vi "test - clear JKI String Queue Error.vi"(8 "error in (no error)":errorcluster, 11 "TestCase in":refnum<class "testcase-Basic-Function.lvclass">) -> (0 "error out":errorcluster, 3 "TestCase out":refnum<class "testcase-Basic-Function.lvclass">)   [LabVIEW 2017, in "testcase-Basic-Function.lvclass"]
uses:
  testcase-Basic-Function.lvclass
  161a5074-68cb-42ac-bbbd-290e101bf616.vi
  src/user.lib/_NEVSTOP/Communicable State Machine(CSM)/AdvanceAPI/CSM - Revert Arguments-Safe String.vi
  src/user.lib/_NEVSTOP/Communicable State Machine(CSM)/_Support/Common/Trim Single line Text.vi
  src/user.lib/_NEVSTOP/Communicable State Machine(CSM)/AdvanceAPI/CSM - Make String Arguments Safe.vi
  src/user.lib/_NEVSTOP/Communicable State Machine(CSM)/AdvanceAPI/CSM - Break Down Multiple States String.vi
  src/user.lib/_NEVSTOP/Communicable State Machine(CSM)/AdvanceAPI/CSM - Compact Multiple States.vi
  src/user.lib/_NEVSTOP/Communicable State Machine(CSM)/AdvanceAPI/CSM - Keywords.vi
  <vilib>/addons/_JKI Toolkits/VI Tester/TestCase.llb/TestCase.lvclass
  src/user.lib/_NEVSTOP/Communicable State Machine(CSM)/Communicable State Machine.lvlib
  C:/Program Files (x86)/National Instruments/LabVIEW 2017/vi.lib/addons/_JKI Toolkits/VI Tester/TestCase.llb/TestCase.lvclass
panel:
  out "error in CSM":errorcluster
  in  "x":bool
  out "error for return":errorcluster
  out "State History":string
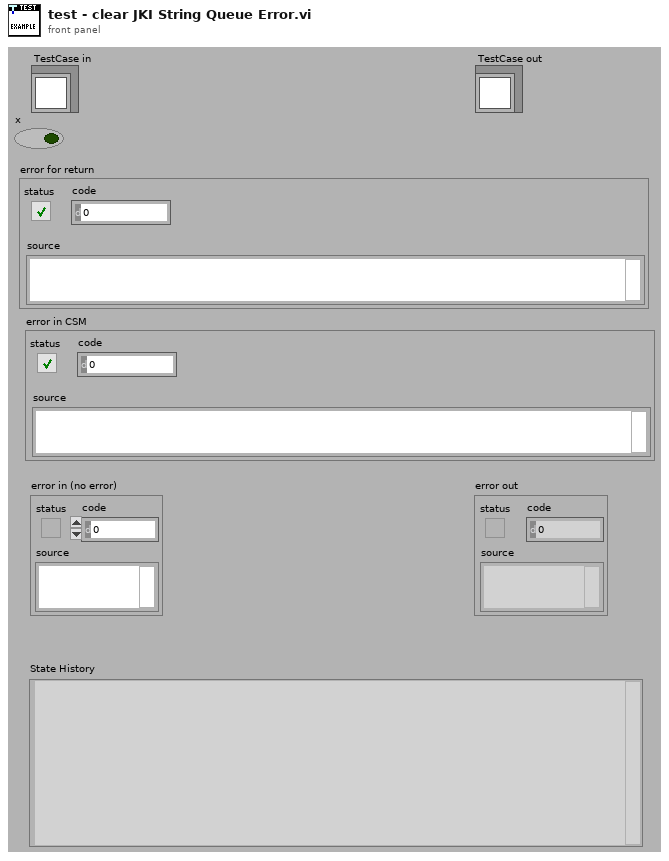
[diagram p1: front panel]
types:
  T1 = enum32{"Invalid", "Standard", "Closed", "Hidden", "Minimized", "Maximized"}
  T2 = enum32{"invalid app kind", "Development System", "Run Time System", "Student Edition", "Embedded LabVIEW", "Evaluation", "Custom"}
  T3 = typedef "Communicable State Machine.lvlib/_CSM_Response Source Message.ctl" = cluster{"‘State":string, "’Arguments":string, "’Error":errorcluster}
  T4 = cluster{"Current VI Reference":refnum<vi>, "Close Panel on Exit?":bool}
  T5 = cluster{"Core":cluster{"Current VI Reference":refnum<vi>, "Close Panel on Exit?":bool}, "Your Boolean data":bool, "Your string data":string}
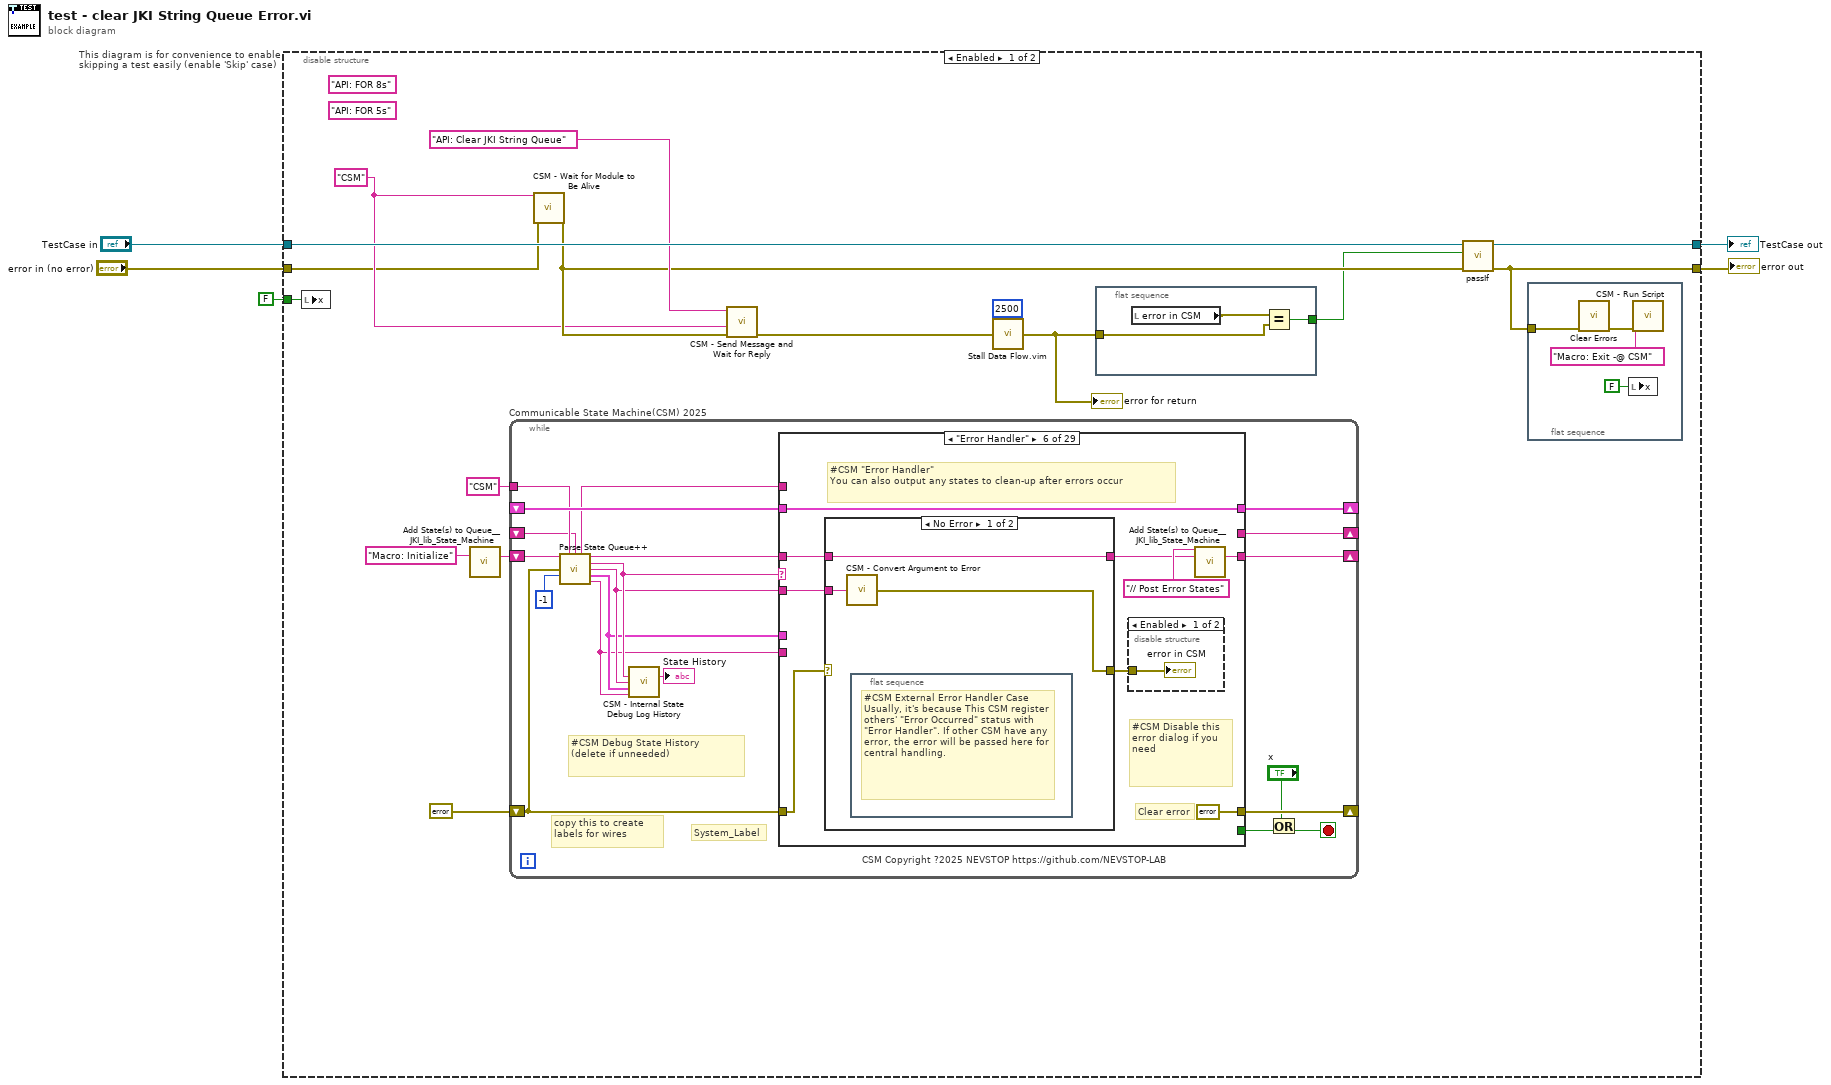
[diagram p0: block diagram]
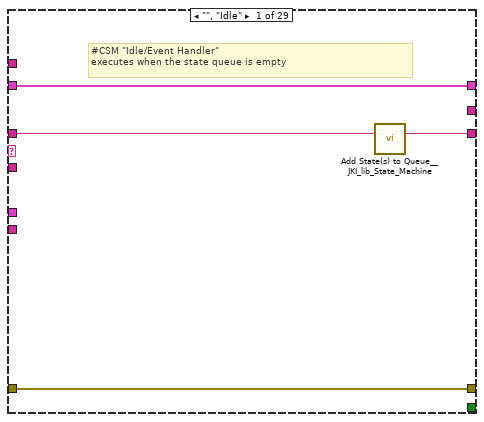
[diagram p2: hidden frame]
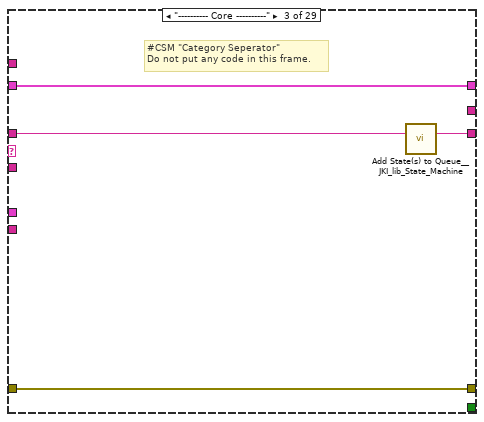
[diagram p4: hidden frame]
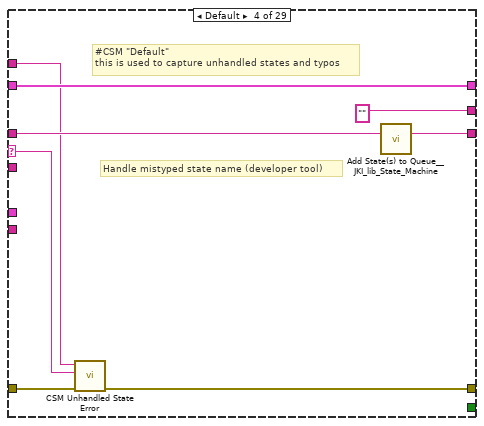
[diagram p5: hidden frame]
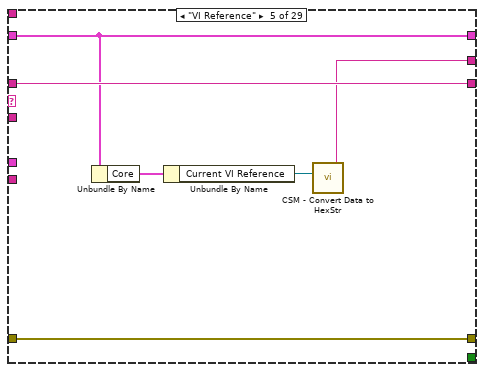
[diagram p6: hidden frame]
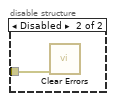
[diagram p7: hidden frame]
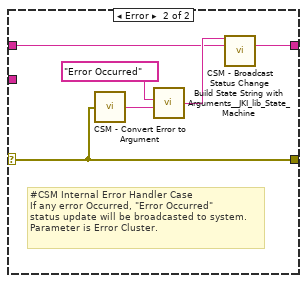
[diagram p8: hidden frame]
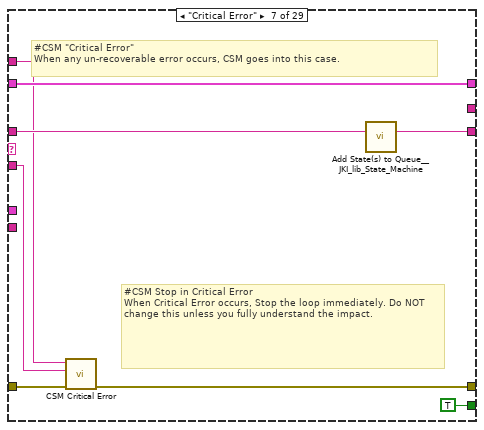
[diagram p9: hidden frame]
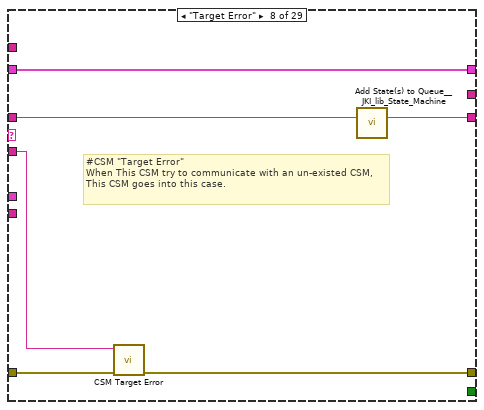
[diagram p10: hidden frame]
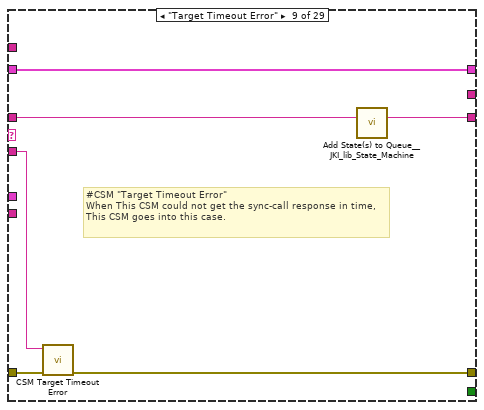
[diagram p11: hidden frame]
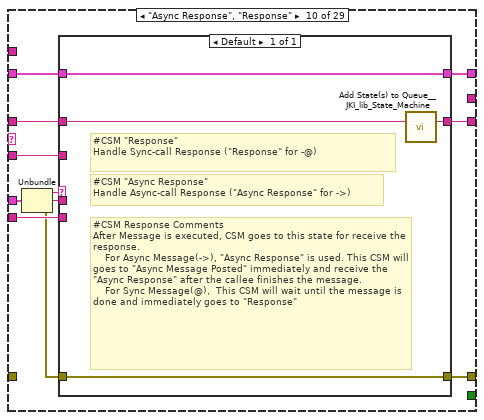
[diagram p12: hidden frame]
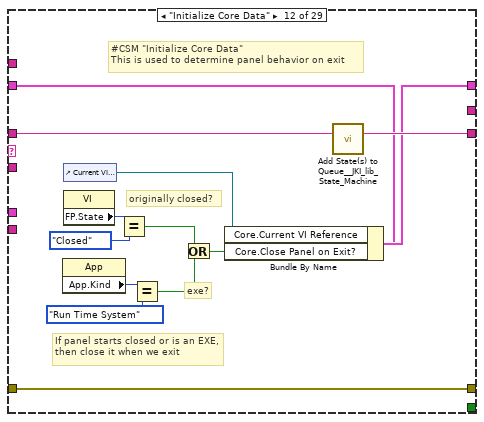
[diagram p14: hidden frame]
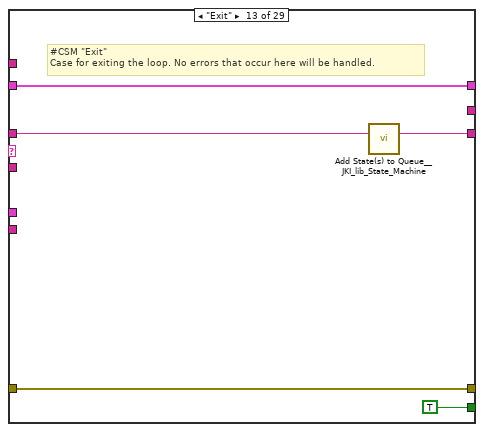
[diagram p15: hidden frame]
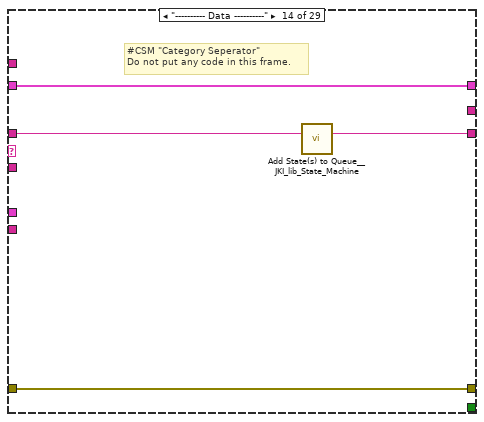
[diagram p16: hidden frame]
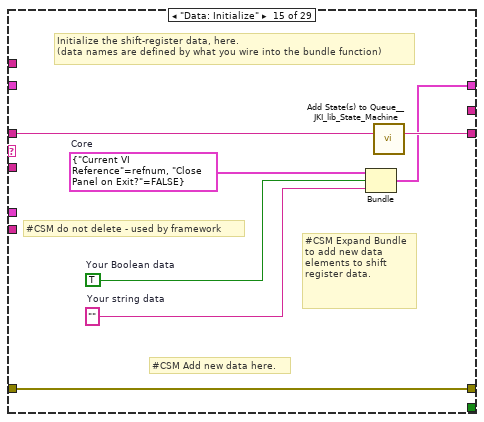
[diagram p17: hidden frame]
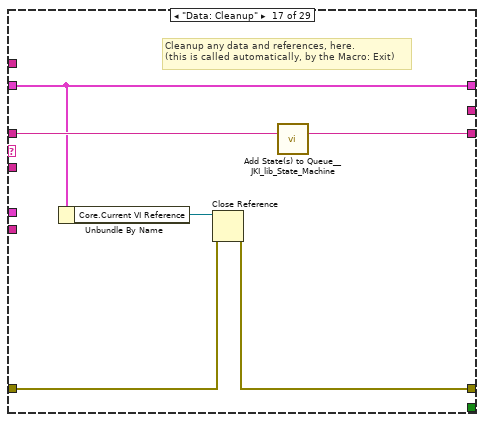
[diagram p19: hidden frame]
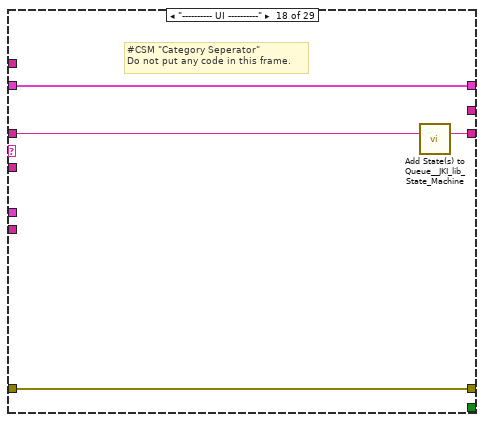
[diagram p20: hidden frame]
diagram:
  n1 = disable-structure "This diagram is for convenience to enable skipping a test easily (enable 'Skip' case)" shown="Enabled" {
    disable-tunnel: "TestCase in" -> [w15 w300]
    disable-tunnel: [w17 w298] -> w2
    disable-tunnel: [w16 w299] -> w4
    disable-tunnel: "error in (no error)" -> [w11 w297]
    disable-tunnel: FALSE ("x") -> [w8 _]
    frame Enabled {
      (unwired) "API: FOR 8s" ("State")
      (unwired) "API: FOR 5s" ("State")
      w12 = "CSM" ("Name(\"\" to use uuid)")
      n2 = local write "x"(w8) -> ()
      n3 = call <vilib>:"Add State(s) to Queue__JKI_lib_State_Machine.vi"("State(s) in (\"\")"="Macro: Initialize" ("Init State(\"Macro: Initialize\")")) -> ("States Out"=w21:string)  [unwired: 14 in]
      n4 = while "Communicable State Machine(CSM) 2025" {
        shift-right: [w43] -> _
        shift-left: _ -> [w42]
        shift-right: [w46] -> _
        shift-left: errorcluster {"status"=FALSE, "code"=0, "source"=""} ("error out") -> [w41]
        shift-right: [w45] -> _
        shift-left: w21 -> [w47]
        tunnel: "CSM" ("Name(\"\" to use uuid)") -> [w39]
        shift-right: [w40] -> _
        shift-left: _ -> [w33]
        stop <- w30 stop-if-true
        # "#CSM Debug State History\n(delete if unneeded)"
        # "copy this to create labels for wires"
        # "System_Label"
        # "CSM Copyright ?2025 NEVSTOP https://github.com/NEVSTOP-LAB"
        n5 = call "Parse State Queue++.vi"("State Queue"=w47, "Name(\"\" to use uuid)"=w39, "Response Arguments"=w33, "Previous Error"=w41, "Dequeue Timeout(0ms)"=-1 ("Timeout")) -> ("Name Used"=w34:string, "Remaining States"=w48:string, "Current State"=w38:string, "Arguments"=w37:string, ">> Response Source Message >>"=w36:T3, ">> Source CSM >>"=w35:string)  [unwired: 5 in]
        n6 = call "CSM - Internal State Debug Log History.vi"("State"=w38, "Arguments (\"\")"=w37, ">> Response Source Message >>"=w36, "Source (\"\")"=w35) -> ("Debug Log"=→"State History":string)  [unwired: 11 in]
        n7 = case shown="\"Error Handler\"" w38 {
          selector: w38 -> [_ _ _ w62 _ _ _ _ _ _ _ _ _ _ _ _ _ _ _ _ _ _ _ _ _ _ _ _ _]
          tunnel: w48 -> [w49 w54 w59 w66 w72 w78 w99 w105 w111 w119 w130 w144 w149 w153 w160 w162 w169 w173 w177 w183 w198 w267 w272 w279 w281 _ w288 w292 w296]
          tunnel: w37 -> [_ _ _ _ _ w77 w95 w104 w109 w118 _ _ _ _ _ _ _ _ _ w178 w192 _ _ _ _ _ _ _ _]
          tunnel: w42 -> [w50 w53 w56 w64 w71 w81 w100 w106 w112 w121 w129 w137 w147 w150 _ w161 w164 w170 w175 w181 w194 w264 w269 w276 w280 w283 w285 w289 w293]
          tunnel: [w51 w55 w57 w60 w73 errorcluster {"status"=FALSE, "code"=0, "source"=""} ("error out") w96 w102 w108 w124 w131 w141 w146 w151 w157 w163 w165 w171 w174 w179 w195 w265 w270 w277 w282 w284 w286 w290 w294] -> w46
          tunnel: w41 -> [w51 w55 w57 w67 w73 w79 w101 w103 w110 _ w131 w141 w146 w151 w157 w163 w166 w171 w174 w180 w196 w265 w270 w277 w282 w284 w286 w290 w294]
          tunnel: [w52 w54 w58 w65 w72 w74 w98 w107 w113 w120 w130 w143 w148 w152 w159 w162 w168 w172 w176 w182 w197 w266 w271 w278 w281 _ w287 w291 w295] -> w45
          tunnel: [_ _ _ _ _ _ TRUE _ _ _ _ _ TRUE _ _ _ _ _ _ _ _ _ _ _ _ _ _ _ _] -> w44
          tunnel: [w50 w53 w56 w64 w71 w81 w100 w106 w112 w122 w129 w142 w147 w150 w158 w161 w164 w170 w175 w181 w194 w264 w269 w276 w280 w283 w285 w289 w293] -> w43
          tunnel: w35 -> [_ _ _ _ _ _ _ _ _ w116 _ _ _ _ _ _ _ _ _ _ _ _ _ _ _ _ _ _ _]
          tunnel: w36 -> [_ _ _ _ _ _ _ _ _ w123 _ _ _ _ _ _ _ _ _ _ _ _ _ _ _ _ _ _ _]
          tunnel: [_ _ _ "" w68 _ _ _ _ _ _ _ _ _ _ _ _ _ _ _ _ _ _ _ _ _ _ _ _] -> w40
          tunnel: w34 -> [_ _ _ w61 _ _ w94 _ _ _ _ _ _ _ _ _ _ _ _ _ _ _ _ _ _ _ _ _ _]
          frame "", "Idle" {
            # "#CSM \"Idle/Event Handler\"\nexecutes when the state queue is empty"
            n8 = call <vilib>:"Add State(s) to Queue__JKI_lib_State_Machine.vi"("State(s) in (\"\")"=w49) -> ("States Out"=w52:string)  [unwired: 14 in]
          }
          frame "CSM Documentation" {
            # "#CSM README FIRST\n\nCommunicable State Machine(CSM) is a LabVIEW application framework that builds upon JKI State Machine(JKISM). It follows the pattern of JKISM and extends the keywords to describe message communication between modules, including concepts such as Sync-Message, Async-Message, Subscription/Unsubscription of status - essential elements for creating reusable code modules. For more information, please visit the CSM wiki: https://nevstop-lab.github.io/CSM-Wiki/\n\nFor instructions on JKI State Machine, visit: http://jki.net/state-machine/\nFor information about CSM, visit: https://github.com/NEVSTOP-LAB"
            # "#CSM \"Documentation\"\nCase for holding CSM Documenation"
          }
          frame "---------- Core ----------" {
            # "#CSM \"Category Seperator\"\nDo not put any code in this frame."
            n9 = call <vilib>:"Add State(s) to Queue__JKI_lib_State_Machine.vi"("State(s) in (\"\")"=w59) -> ("States Out"=w58:string)  [unwired: 14 in]
          }
          frame Default {
            # "#CSM \"Default\"\nthis is used to capture unhandled states and typos"
            # "Handle mistyped state name (developer tool)"
            n10 = call "CSM Unhandled State Error.vi"("error in (no error)"=w67, "Current State"=w62, "CSM Name"=w61) -> ("error out"=w60:errorcluster)  [unwired: 8 in]
            n11 = call <vilib>:"Add State(s) to Queue__JKI_lib_State_Machine.vi"("State(s) in (\"\")"=w66) -> ("States Out"=w65:string)  [unwired: 14 in]
          }
          frame "VI Reference" {
            n12 = Unbundle By Name(w71) -> ("Core"=w70:T4)
            n13 = Unbundle By Name(w70) -> ("Current VI Reference"=w69:refnum<vi>)
            n14 = call "CSM - Convert Data to HexStr.vi"("Variant"=w69) -> ("HEX String (0-9,A-F)"=w68:string)  [unwired: 8 in]
          }
          frame "Error Handler" {
            # "#CSM Disable this error dialog if you need"
            # "#CSM \"Error Handler\"\nYou can also output any states to clean-up after errors occur"
            # "Clear error"
            n15 = case shown="No Error" w79 {
              selector: w79 -> [_ w88]
              tunnel: [w87 w90] -> w75
              tunnel: w78 -> [w87 w89]
              tunnel: w77 -> [w86 _]
              tunnel: [w85 w88] -> w80
              frame No Error {
                n16 = call "CSM - Convert Argument to Error.vi"("Argument"=w86) -> ("error"=w85:errorcluster)  [unwired: 4 in]
                n17 = flat-sequence {
                  frame #0 {
                    # "#CSM External Error Handler Case\nUsually, it's because This CSM register others' \"Error Occurred\" status with \"Error Handler\". If other CSM have any error, the error will be passed here for central handling."
                  }
                }
              }
              frame Error {
                # "#CSM Internal Error Handler Case \nIf any error Occurred, \"Error Occurred\" \nstatus update will be broadcasted to system.\nParameter is Error Cluster."
                n18 = call "CSM - Convert Error to Argument.vi"("error"=w88) -> ("Argument"=w92:string)  [unwired: 4 in]
                n19 = call <vilib>:"Build State String with Arguments__JKI_lib_State_Machine.vi"("Arguments (\"\")"=w92, "State"="Error Occurred" ("Status with Arguments")) -> ("State with Arguments"=w91:string)  [unwired: 4 in]
                n20 = call "CSM - Broadcast Status Change.vi"("Status with Arguments"=w91, "State Queue"=w89) -> ("Remaining States"=w90:string)  [unwired: 13 in]
              }
            }
            n21 = disable-structure shown="Enabled" {
              disable-tunnel: w80 -> [w83 w84]
              frame Enabled {
                "error in CSM" <- w83
              }
              frame Disabled {
                n22 = call <vilib>:"Clear Errors.vi"("error in (no error)"=w84) -> ()  [unwired: 5 in, 2 out]
              }
            }
            n23 = call <vilib>:"Add State(s) to Queue__JKI_lib_State_Machine.vi"("State(s) in Front (\"\")"="// Post Error States", "State(s) in (\"\")"=w75) -> ("States Out"=w74:string)  [unwired: 13 in]
          }
          frame "Critical Error" {
            # "#CSM Stop in Critical Error\nWhen Critical Error occurs, Stop the loop immediately. Do NOT change this unless you fully understand the impact."
            # "#CSM \"Critical Error\"\nWhen any un-recoverable error occurs, CSM goes into this case."
            n24 = call "CSM Critical Error.vi"("error in (no error)"=w101, "Arugments(as Reason)"=w95, "CSM Name"=w94) -> ("error out"=w96:errorcluster)  [unwired: 8 in]
            n25 = call <vilib>:"Add State(s) to Queue__JKI_lib_State_Machine.vi"("State(s) in (\"\")"=w99) -> ("States Out"=w98:string)  [unwired: 14 in]
          }
          frame "Target Error" {
            # "#CSM \"Target Error\"\nWhen This CSM try to communicate with an un-existed CSM, This CSM goes into this case."
            n26 = call "CSM Target Error.vi"("error in (no error)"=w103, "Arguments(as CSM Name)"=w104) -> ("error out"=w102:errorcluster)  [unwired: 9 in]
            n27 = call <vilib>:"Add State(s) to Queue__JKI_lib_State_Machine.vi"("State(s) in (\"\")"=w105) -> ("States Out"=w107:string)  [unwired: 14 in]
          }
          frame "Target Timeout Error" {
            # "#CSM \"Target Timeout Error\"\nWhen This CSM could not get the sync-call response in time, This CSM goes into this case."
            n28 = call "CSM Target Timeout Error.vi"("error in (no error)"=w110, "Arguments(as CSM Name)"=w109) -> ("error out"=w108:errorcluster)  [unwired: 9 in]
            n29 = call <vilib>:"Add State(s) to Queue__JKI_lib_State_Machine.vi"("State(s) in (\"\")"=w111) -> ("States Out"=w113:string)  [unwired: 14 in]
          }
          frame "Async Response", "Response" {
            n30 = Unbundle(w123) -> ("‘State"=w117:string, "’Arguments"=w115:string, "’Error"=w114:errorcluster)
            n31 = case shown="Default" w117 {
              tunnel: [w128] -> w124
              tunnel: w114 -> [w128]
              tunnel: [w127] -> w122
              tunnel: w121 -> [w127]
              tunnel: [w125] -> w120
              tunnel: w119 -> [w126]
              tunnel: w118 -> [_]
              tunnel: w116 -> [_]
              tunnel: w115 -> [_]
              frame Default {
                # "#CSM Response Comments\nAfter Message is executed, CSM goes to this state for receive the response.\n    For Async Message(->), \"Async Response\" is used. This CSM will goes to \"Async Message Posted\" immediately and receive the \"Async Response\" after the callee finishes the message.\n    For Sync Message(@),  This CSM will wait until the message is done and immediately goes to \"Response\""
                # "#CSM \"Async Response\"\nHandle Async-call Response (\"Async Response\" for ->)"
                # "#CSM \"Response\"\nHandle Sync-call Response (\"Response\" for -@)"
                n32 = call <vilib>:"Add State(s) to Queue__JKI_lib_State_Machine.vi"("State(s) in (\"\")"=w126) -> ("States Out"=w125:string)  [unwired: 14 in]
              }
            }
          }
          frame "Async Message Posted" {
            # "#CSM \"Async Message Posted\"\nAfter Async Message is posted (-> or ->| ), CSM goes to this state for post-action.\nYou can use Argument - State to tell which Async Message is called."
          }
          frame "Initialize Core Data" {
            # "#CSM \"Initialize Core Data\"\nThis is used to determine panel behavior on exit"
            # "originally closed?"
            # "exe?"
            # "If panel starts closed or is an EXE, then close it when we exit"
            n33 = property class="App"() -> ("App.Kind"=w140:T2)  [unwired: 2 in, 2 out]
            n34 = control-ref of="Current VI Reference"() -> (w135:refnum<vi>)
            n35 = property class="VI"() -> ("FP.State"=w134:T1)  [unwired: 2 in, 2 out]
            n36 = Equal?(x=w134, y=T1."Closed" ("Front Panel Window:State")) -> (x = y?=w132:bool)
            n37 = Equal?(x=w140, y=T2."Run Time System" ("Application:Kind")) -> (x = y?=w138:bool)
            n38 = Or(x=w132, y=w138) -> (x .or. y?=w136:bool)
            n39 = Bundle By Name(cluster=w137, "Core.Current VI Reference"=w135, "Core.Close Panel on Exit?"=w136) -> (w142:T5)
            n40 = call <vilib>:"Add State(s) to Queue__JKI_lib_State_Machine.vi"("State(s) in (\"\")"=w144) -> ("States Out"=w143:string)  [unwired: 14 in]
          }
          frame "Exit" {
            # "#CSM \"Exit\"\nCase for exiting the loop. No errors that occur here will be handled."
            n41 = call <vilib>:"Add State(s) to Queue__JKI_lib_State_Machine.vi"("State(s) in (\"\")"=w149) -> ("States Out"=w148:string)  [unwired: 14 in]
          }
          frame "---------- Data ----------" {
            # "#CSM \"Category Seperator\"\nDo not put any code in this frame."
            n42 = call <vilib>:"Add State(s) to Queue__JKI_lib_State_Machine.vi"("State(s) in (\"\")"=w153) -> ("States Out"=w152:string)  [unwired: 14 in]
          }
          frame "Data: Initialize" {
            w154 = T4 {"Current VI Reference"=refnum, "Close Panel on Exit?"=FALSE}  # Core
            w156 = TRUE  # Your Boolean data
            w155 = ""  # Your string data
            # "#CSM do not delete - used by framework"
            # "#CSM Expand Bundle to add new data elements to shift register data."
            # "#CSM Add new data here."
            # "Initialize the shift-register data, here.\n(data names are defined by what you wire into the bundle function)"
            n43 = Bundle("Core"=w154, "Your Boolean data"=w156, "Your string data"=w155) -> (w158:T5)  [unwired: 1 in]
            n44 = call <vilib>:"Add State(s) to Queue__JKI_lib_State_Machine.vi"("State(s) in (\"\")"=w160) -> ("States Out"=w159:string)  [unwired: 14 in]
          }
          frame "Data: Update Indicators" {
          }
          frame "Data: Cleanup" {
            # "Cleanup any data and references, here.\n(this is called automatically, by the Macro: Exit)"
            n45 = Unbundle By Name(w164) -> ("Core.Current VI Reference"=w167:refnum<vi>)
            n46 = Close Reference(reference=w167, error in (no error)=w166) -> (error out=w165:errorcluster)
            n47 = call <vilib>:"Add State(s) to Queue__JKI_lib_State_Machine.vi"("State(s) in (\"\")"=w169) -> ("States Out"=w168:string)  [unwired: 14 in]
          }
          frame "---------- UI ----------" {
            # "#CSM \"Category Seperator\"\nDo not put any code in this frame."
            n48 = call <vilib>:"Add State(s) to Queue__JKI_lib_State_Machine.vi"("State(s) in (\"\")"=w173) -> ("States Out"=w172:string)  [unwired: 14 in]
          }
          frame "UI: Initialize" {
            # "#CSM \"UI: Initialize\"\nInitialize the User Interface, here.\n(this is called automatically, by the Macro: Init)"
            n49 = call <vilib>:"Add State(s) to Queue__JKI_lib_State_Machine.vi"("State(s) in (\"\")"=w177) -> ("States Out"=w176:string)  [unwired: 14 in]
          }
          frame "UI: Cursor Set" {
            # "#CSM \"UI: Cursor Set\"\nSet and Unset Cursor Busy.\n(Usage: \"UI: Cursor Set >> Busy|Idle\")"
            # "Argument"
            n50 = disable-structure shown="TARGET_TYPE!=Windows" {
              disable-tunnel: w180 -> [w186 w191]
              disable-tunnel: [w185 w191] -> w179
              disable-tunnel: w178 -> [w184 _]
              frame condition #0 (active) {
                n51 = case shown="\"Idle\", Default" w184 {
                  tunnel: w186 -> [w188 w190]
                  tunnel: [w187 w189] -> w185
                  frame "Idle", Default {
                    n52 = call <vilib>:"Unset Busy.vi"("error in (no error)"=w188) -> ("error out"=w187:errorcluster)  [unwired: 10 in]
                  }
                  frame "Busy" {
                    n53 = call <vilib>:"Set Busy.vi"("error in (no error)"=w190) -> ("error out"=w189:errorcluster)  [unwired: 9 in, 1 out]
                  }
                }
              }
              frame condition #1 {
              }
            }
            n54 = call <vilib>:"Add State(s) to Queue__JKI_lib_State_Machine.vi"("State(s) in (\"\")"=w183) -> ("States Out"=w182:string)  [unwired: 14 in]
          }
          frame "UI: Front Panel State" {
            # "#CSM \"UI: Front Panel State\"\nSet Front Panel Open or Closed\n(Usage: \"UI: Front Panel State >> Open|Close\")"
            # "Argument"
            n55 = Unbundle By Name(w194) -> ("Core.Current VI Reference"=w193:refnum<vi>)
            n56 = call <vilib>:"Add State(s) to Queue__JKI_lib_State_Machine.vi"("State(s) in (\"\")"=w198) -> ("States Out"=w197:string)  [unwired: 14 in]
            n57 = case shown="\"Close\", \"Closed\"" w192 {
              tunnel: w196 -> [w204 w219 w230 w243 w256]
              tunnel: [w206 w220 w232 w245 w258] -> w195
              tunnel: w193 -> [w205 w217 w231 w244 w257]
              frame "Open", "Standard", Default {
                w199 = T1."Standard" ("State")
                n58 = property class="VI"(reference=w205, error in=w204) -> (reference out=w202:refnum<vi>, error out=w203:errorcluster, "FP.State"=w201:T1)
                n59 = Not Equal?(x=w201, y=w199) -> (x != y?=w200:bool)
                n60 = case shown="True" w200 {
                  tunnel: [w210 w212] -> w206
                  tunnel: w203 -> [w209 w212]
                  tunnel: w202 -> [w208 _]
                  tunnel: w199 -> [w207 _]
                  frame True {
                    n61 = invoke class="VI" method="FP.Open"(reference=w208, error in=w209, "Activate"=TRUE, "State"=w207) -> (error out=w210:errorcluster)  [unwired: 1 in, 4 out]
                  }
                  frame False {
                  }
                }
              }
              frame "Close", "Closed" {
                n62 = property class="VI"(reference=w217, error in=w219) -> (reference out=w216:refnum<vi>, error out=w218:errorcluster, "FP.State"=w214:T1)
                n63 = Not Equal?(x=w214, y=T1."Closed" ("Front Panel Window:State")) -> (x != y?=w213:bool)
                n64 = case shown="False" w213 {
                  tunnel: [w221 w224] -> w220
                  tunnel: w218 -> [w221 w223]
                  tunnel: w216 -> [_ w222]
                  frame False {
                  }
                  frame True {
                    n65 = invoke class="VI" method="FP.Close"(reference=w222, error in=w223) -> (error out=w224:errorcluster)  [unwired: 1 in, 2 out]
                  }
                }
              }
              frame "Hidden", "Hide" {
                w225 = T1."Hidden" ("State")
                n66 = property class="VI"(reference=w231, error in=w230) -> (reference out=w228:refnum<vi>, error out=w229:errorcluster, "FP.State"=w227:T1)
                n67 = Not Equal?(x=w227, y=w225) -> (x != y?=w226:bool)
                n68 = case shown="True" w226 {
                  tunnel: [w236 w237] -> w232
                  tunnel: w229 -> [w235 w237]
                  tunnel: w228 -> [w234 _]
                  tunnel: w225 -> [w233 _]
                  frame True {
                    n69 = invoke class="VI" method="FP.Open"(reference=w234, error in=w235, "State"=w233) -> (error out=w236:errorcluster)  [unwired: 2 in, 4 out]
                  }
                  frame False {
                  }
                }
              }
              frame "Minimize", "Minimized" {
                w238 = T1."Minimized" ("State")
                n70 = property class="VI"(reference=w244, error in=w243) -> (reference out=w241:refnum<vi>, error out=w242:errorcluster, "FP.State"=w240:T1)
                n71 = Not Equal?(x=w240, y=w238) -> (x != y?=w239:bool)
                n72 = case shown="True" w239 {
                  tunnel: [w249 w250] -> w245
                  tunnel: w242 -> [w248 w250]
                  tunnel: w241 -> [w247 _]
                  tunnel: w238 -> [w246 _]
                  frame True {
                    n73 = invoke class="VI" method="FP.Open"(reference=w247, error in=w248, "State"=w246) -> (error out=w249:errorcluster)  [unwired: 2 in, 4 out]
                  }
                  frame False {
                  }
                }
              }
              frame "Maximize", "Maximized" {
                w251 = T1."Maximized" ("State")
                n74 = property class="VI"(reference=w257, error in=w256) -> (reference out=w254:refnum<vi>, error out=w255:errorcluster, "FP.State"=w253:T1)
                n75 = Not Equal?(x=w253, y=w251) -> (x != y?=w252:bool)
                n76 = case shown="True" w252 {
                  tunnel: [w262 w263] -> w258
                  tunnel: w255 -> [w261 w263]
                  tunnel: w254 -> [w260 _]
                  tunnel: w251 -> [w259 _]
                  frame True {
                    n77 = invoke class="VI" method="FP.Open"(reference=w260, error in=w261, "State"=w259) -> (error out=w262:errorcluster)  [unwired: 2 in, 4 out]
                  }
                  frame False {
                  }
                }
              }
            }
          }
          frame "---------- Macro ----------" {
            # "#CSM \"Category Seperator\"\nDo not put any code in this frame."
            n78 = call <vilib>:"Add State(s) to Queue__JKI_lib_State_Machine.vi"("State(s) in (\"\")"=w267) -> ("States Out"=w266:string)  [unwired: 14 in]
          }
          frame "Macro: Initialize" {
            # "#CSM \"Macro: Initialize\"\nInitialization Macro (This is called once, when the VI starts)"
            n79 = call <vilib>:"Add State(s) to Queue__JKI_lib_State_Machine.vi"("State(s) in Front (\"\")"="Data: Initialize\nInitialize Core Data\nData: Update Indicators", "State(s) in (\"\")"=w272) -> ("States Out"=w271:string)  [unwired: 13 in]
          }
          frame "Macro: Exit" {
            # "#CSM \"Macro: Exit\"\nExit Macro (This is called once, when the VI exits)"
            n80 = call <vilib>:"Add State(s) to Queue__JKI_lib_State_Machine.vi"("State(s) in Front (\"\")"="//Exit Sub-Modules ", "State(s) at Back (\"\")"="Data: Cleanup\nExit") -> ("States Out"=w274:string)  [unwired: 13 in]
            n81 = call <vilib>:"Add State(s) to Queue__JKI_lib_State_Machine.vi"("State(s) in Front (\"\")"=w274, "State(s) in (\"\")"=w279) -> ("States Out"=w278:string)  [unwired: 13 in]
          }
          frame "---------- API ----------" {
            # "#CSM \"Category Seperator\"\nDo not put any code in this frame."
          }
          frame "API: Clear JKI String Queue" {
          }
          frame "---------- Action ----------" {
            # "#CSM \"Category Seperator\"\nDo not put any code in this frame."
            n82 = call <vilib>:"Add State(s) to Queue__JKI_lib_State_Machine.vi"("State(s) in (\"\")"=w288) -> ("States Out"=w287:string)  [unwired: 14 in]
          }
          frame "Action: action1" {
            # "#CSM \"Internal State\"\nThis category is used for holding internal states"
            n83 = call <vilib>:"Add State(s) to Queue__JKI_lib_State_Machine.vi"("State(s) in (\"\")"=w292) -> ("States Out"=w291:string)  [unwired: 14 in]
          }
          frame "Action: action2" {
            # "#CSM \"Internal State\"\nThis category is used for holding internal states"
            n84 = call <vilib>:"Add State(s) to Queue__JKI_lib_State_Machine.vi"("State(s) in (\"\")"=w296) -> ("States Out"=w295:string)  [unwired: 14 in]
          }
        }
        n85 = Or(x="x", y=w44) -> (x .or. y?=w30:bool)
      }
      n86 = call "CSM - Wait for Module to Be Alive.vi"("CSM Name"=w12, "error in (no error)"=w11) -> ("error out"=w13:errorcluster)  [unwired: 11 in, 2 out]
      n87 = call "CSM - Send Message and Wait for Reply.vi"("Error In (no error)"=w13, "Target Module"=w12, "State"="API: Clear JKI String Queue") -> ("error out"=w10:errorcluster)  [unwired: 6 in, 2 out]
      n88 = call "Stall Data Flow.vim"("value in"=w10, "milliseconds to wait"=u32 2500) -> ("value out"=w7:errorcluster)  [unwired: 1 out]
      "error for return" <- w7
      n89 = flat-sequence {
        tunnel: [w24] -> w9
        tunnel: w7 -> [w23]
        frame #0 {
          n90 = local read "error in CSM"() -> (w22:errorcluster)
          n91 = Equal?(x=w22, y=w23) -> (x = y?=w24:bool)
        }
      }
      n92 = call-dynamic "passIf.vi"("error in (no error)"=w13, "pass"=w9, "TestCase in"=w15) -> ("error out"=w16:errorcluster, "TestCase out"=w17:refnum<class "testcase-Basic-Function.lvclass">)  [unwired: 7 in]
      n93 = flat-sequence {
        tunnel: w16 -> [w28]
        frame #0 {
          n94 = call <vilib>:"Clear Errors.vi"("error in (no error)"=w28) -> ("error out"=w27:errorcluster)  [unwired: 5 in, 1 out]
          n95 = local write "x"(FALSE ("x")) -> ()
          n96 = call "CSM - Run Script.vi"("CSM Scripts"="Macro: Exit -@ CSM", "error in (no error)"=w27) -> ()  [unwired: 11 in, 3 out]
        }
      }
    }
    frame Disabled {
      # "skip test result while test is under development"
      n97 = call <vilib>:"skip.vi"("error in (no error)"=w297, "TestCase in"=w300) -> ("error out"=w299:errorcluster, "TestCase out"=w298:refnum<class "testcase-Basic-Function.lvclass">)  [unwired: 8 in]
    }
  }
  "error out" <- w4
  "TestCase out" <- w2
